vi "ROI二值面积.vi"(1 "ROI(T3)":T1, 2 "二值化数组":u8[][](array[numeric])) -> (0 "累加值":dbl)   [LabVIEW 2017]
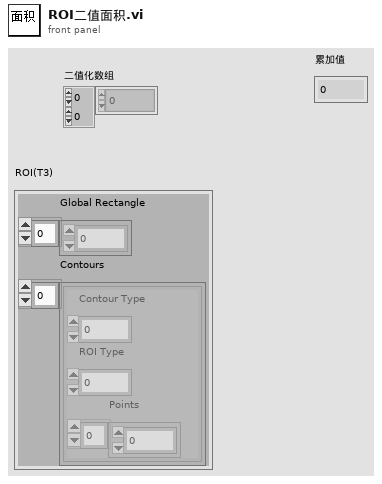
[diagram p1: front panel]
types:
  T1 = cluster{"Global Rectangle":i32[], "Contours":cluster{"Contour Type":u32, "ROI Type":u32, "Points":i32[]}[]}
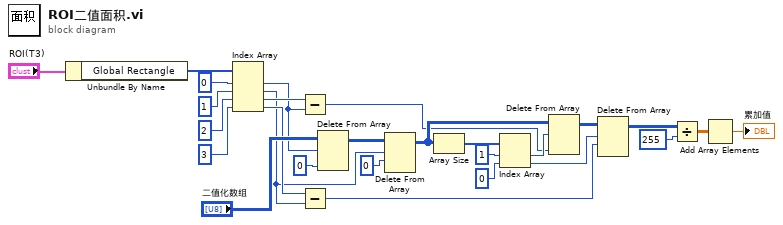
[diagram p0: block diagram]
diagram:
  n1 = Unbundle By Name("ROI(T3)") -> ("Global Rectangle"=w22:i32[])
  n2 = Index Array(array=w22, index #1=0, index #2=1, index #3=2, index #4=3) -> (element #1=w10:i32, element #2=w8:i32, element #3=w11:i32, element #4=w9:i32)
  n3 = Subtract(x=w11, y=w10) -> (x-y=w1:i32)
  n4 = Subtract(x=w9, y=w8) -> (x-y=w2:i32)
  n5 = Delete From Array(array="二值化数组", length=w10, index (col)=0 ("禁用的索引 (列)")) -> (array with subset deleted=w19:u8[][])  [unwired: 1 in, 1 out]
  n6 = Delete From Array(array=w19, length=w8, index (row)=0 ("禁用的索引 (列)")) -> (array with subset deleted=w17:u8[][])  [unwired: 1 in, 1 out]
  n7 = Array Size(array=w17) -> (size(s)=w16:i32[])
  n8 = Index Array(array=w16, index #1=1 ("禁用的索引 (列)"), index #2=0) -> (element #1=w13:i32, element #2=w7:i32)
  n9 = Delete From Array(array=w17, length=w13, index (col)=w1) -> (array with subset deleted=w12:u8[][])  [unwired: 1 in, 1 out]
  n10 = Delete From Array(array=w12, length=w7, index (row)=w2) -> (array with subset deleted=w4:u8[][])  [unwired: 1 in, 1 out]
  n11 = Divide(x=w4, y=255) -> (x/y=w5:dbl[][])
  n12 = Add Array Elements(numeric array=w5) -> (sum=→"累加值":dbl)
